vi "VecBuilder_ArrayBy1Fill.vi"(11 "R Array":dbl[](array[numeric])) -> (3 "Output Vector":T1)   [LabVIEW 2019, in "Trajectory_Library.lvlib"]
doc: "Creates a new LINEAR SYSTEM data cluster with the specified values. \n\n\nInputs: \n - XXX -- XXX.\n\nOutputs:\n - XXX -- XXX."
uses:
  Trajectory_Library.lvlib
  <vilib>/Analysis/Matrix/Datatypes/RealMatrix.ctl
  <vilib>/Analysis/Matrix/NI_Matrix.lvlib
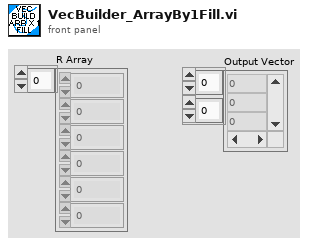
[diagram p1: front panel]
types:
  T1 = typedef "NI_Matrix.lvlib/RealMatrix.ctl" = dbl[][]
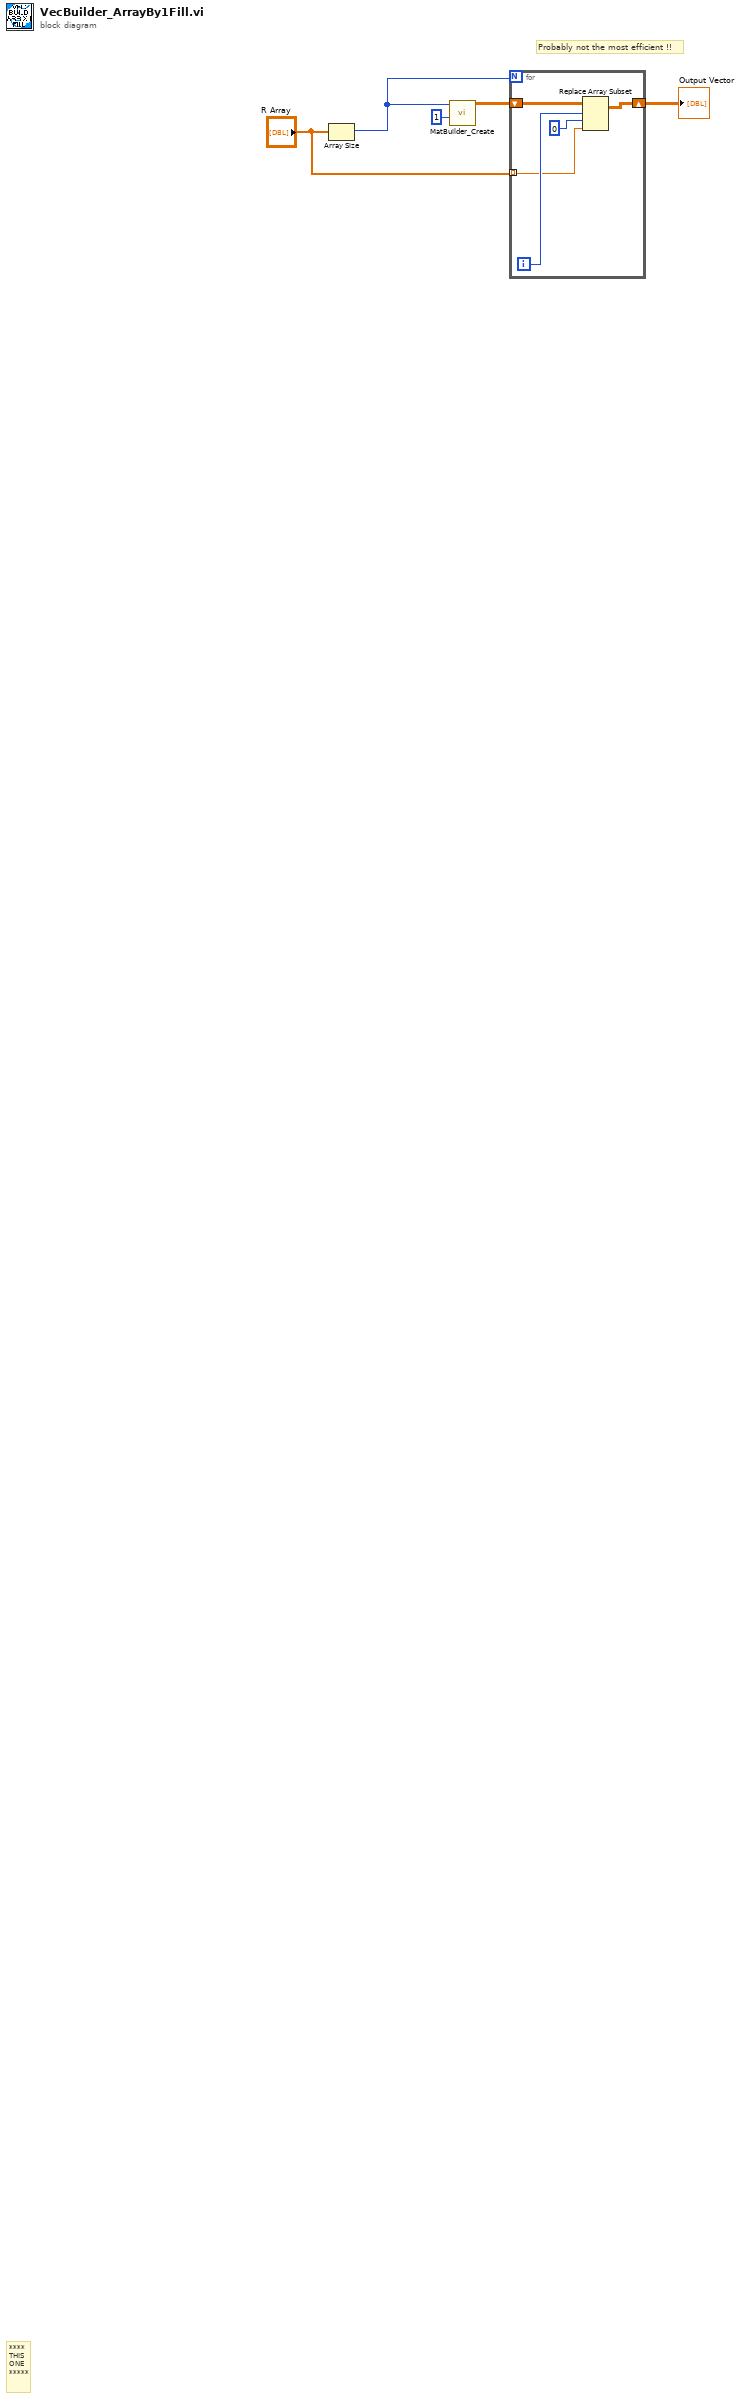
[diagram p0: block diagram]
diagram:
  # "Probably not the most efficient !!"
  # "****\nTHIS\nONE\n*****"
  n1 = Array Size(array="R Array") -> (size(s)=w4:i32)
  n2 = call "MatBuilder_Create.vi"("Columns"=1, "Rows"=w4) -> ("output matrix"=w2:T1)  [unwired: 9 in]
  n3 = for {
    N: w4 -> [_]
    tunnel: "R Array" -> [w6] mode=indexing
    shift-right: [w9] -> w1
    shift-left: w2 -> [w10]
    i -> [w8]
    n4 = Replace Array Subset(array=w10, new element=w6, index (row)=w8, index (col)=0 ("disabled index (col)")) -> (w9:T1)
  }
  "Output Vector" <- w1
